vi "Read Handle.vi"(8 "error in":errorcluster, 11 "Configurable Device in":refnum<class "Configurable Device.lvclass">) -> (0 "error out":errorcluster, 2 "Session Handle":T1, 3 "Configurable Device out":refnum<class "Configurable Device.lvclass">)   [LabVIEW 2018, in "Device.lvlib" / "Configurable Device.lvclass"]
uses:
  Configurable Device.lvclass
  reusable/Session APIs/File Access/Config Data/Config Session.ctl
  reusable/Session APIs/File Access/Config Data/Config Data.lvclass
  Configurable Device.lvclass/Configurable Device.ctl
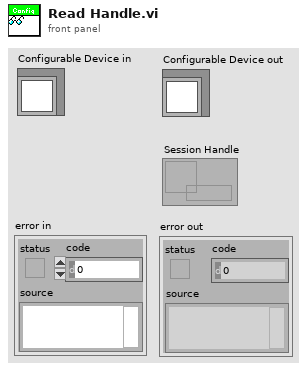
[diagram p1: front panel]
types:
  T1 = typedef "Config Data.lvclass/Config Session.ctl" = refnum<data-value>
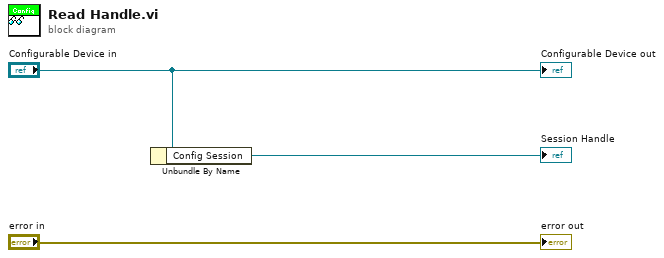
[diagram p0: block diagram]
diagram:
  n1 = Unbundle By Name("Configurable Device in") -> ("Config Session"=→"Session Handle":T1)
  "error out" <- "error in"
  "Configurable Device out" <- "Configurable Device in"
